vi "CompressFile.vi"(8 "error in (no error)":errorcluster, 11 "name":string) -> (0 "error out":errorcluster, 3 "H5 File name":string)   [LabVIEW 2014]
panel:
  out "zip name":string
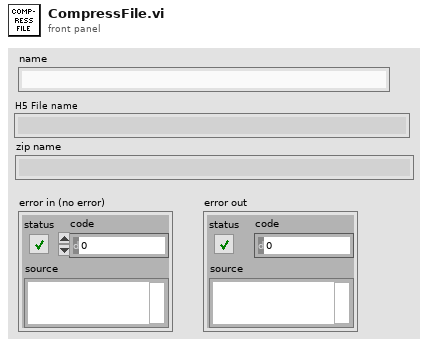
[diagram p1: front panel]
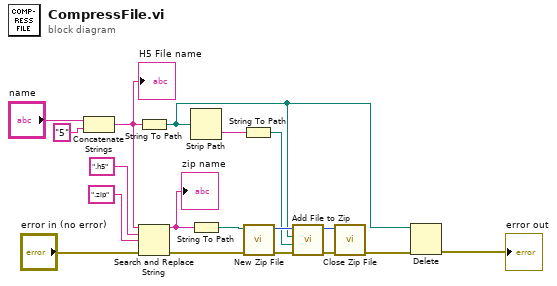
[diagram p0: block diagram]
diagram:
  n1 = Concatenate Strings("name", "5" ("string")) -> (w6:string)
  "H5 File name" <- w6
  n2 = String To Path(string=w6) -> (path=w2:path)
  n3 = Search and Replace String(input string=w6, search string=".h5", replace string=".zip" ("replace string (\"\")"), error in="error in (no error)") -> (result string=w14:string, error out=w8:errorcluster)  [unwired: 4 in, 2 out]
  "zip name" <- w14
  n4 = Strip Path(path=w2) -> (name=w5:string)  [unwired: 1 out]
  n5 = String To Path(string=w14) -> (path=w7:path)
  n6 = String To Path(string=w5) -> (path=w4:path)
  n7 = call <vilib>:"New Zip File.vi"("error in (no error)"=w8, "target"=w7) -> ("error out"=w15:errorcluster, "zip file out"=w16:i64)  [unwired: 3 in, 1 out]
  n8 = call <vilib>:"Add File to Zip.vi"("error in (no error)"=w15, "destination path in zip"=w4, "source file path"=w2, "zip file in"=w16) -> ("error out"=w17:errorcluster, "zip file out"=w18:i64)  [unwired: 6 in]
  n9 = call <vilib>:"Close Zip File.vi"("error in (no error)"=w17, "zip file in"=w18) -> ("error out"=w3:errorcluster)  [unwired: 5 in]
  n10 = Delete(path (use dialog)=w2, error in=w3) -> (error out=→"error out":errorcluster)  [unwired: 3 in, 2 out]
